vi "Intan_SPIbegin.vi"(4 "error in":errorcluster, 7 "VISA resource name":refnum<visa-resource-name>) -> (0 "error out":errorcluster, 2 "Text response":string, 3 "VISA resource name out":refnum<visa-resource-name>)   [LabVIEW 2011]
panel:
  in  "byte count":u32=500
  out "return count":u32
  in  "Teensy event char ('b')":string="b"
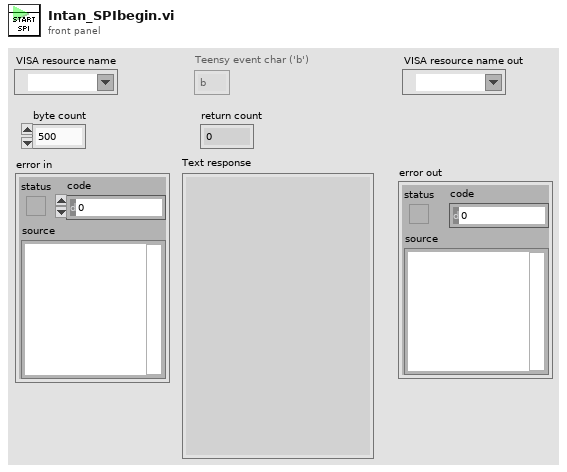
[diagram p1: front panel]
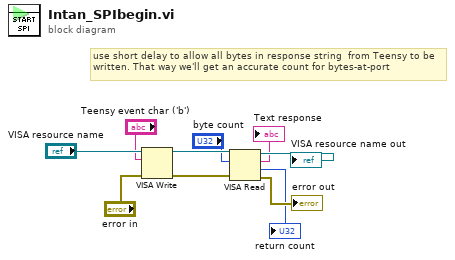
[diagram p0: block diagram]
diagram:
  # "use short delay to allow all bytes in response string  from Teensy to be written. That way we'll get an accurate count for bytes-at-port"
  n1 = VISA Write(VISA resource name="VISA resource name", write buffer="Teensy event char ('b')", error in (no error)="error in") -> (VISA resource name out=w4:refnum<visa-resource-name>, error out=w3:errorcluster)  [unwired: 1 out]
  n2 = VISA Read(VISA resource name=w4, byte count="byte count", error in (no error)=w3) -> (VISA resource name out=→"VISA resource name out":refnum<visa-resource-name>, read buffer=→"Text response":string, return count=→"return count":u32, error out=→"error out":errorcluster)
